vi "ADD Script-Completo.vi"(8 "error in (no error)":errorcluster, 9 "Datos a agregar":string, 11 "VISA resource name":refnum<visa-resource-name>) -> (0 "error out":errorcluster, 3 "VISA resource name out":refnum<visa-resource-name>)   [LabVIEW 2014, in "CAP-USB.lvlib"]
doc: "Genera el codigo para agregar una script\nal CAP-USB enviando todo el codigo por\nserie"
uses:
  CAP-USB.lvlib
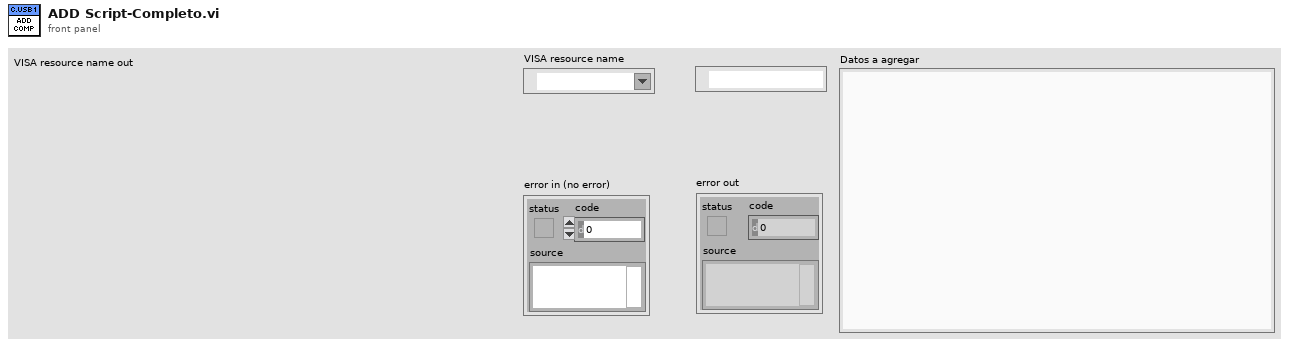
[diagram p1: front panel]
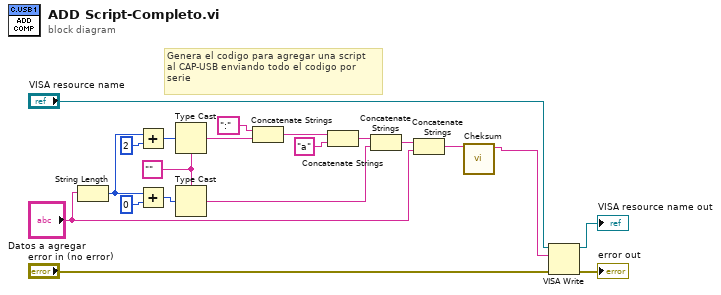
[diagram p0: block diagram]
diagram:
  w14 = "" ("COMANDO (a)")
  # "Genera el codigo para agregar una script\nal CAP-USB enviando todo el codigo por\nserie"
  n1 = String Length(string="Datos a agregar") -> (length=w8:i32)
  n2 = Add(x=w8, y=i8 2) -> (x+y=w15:i8)
  n3 = Add(x=w8, y=i8 0) -> (x+y=w6:i8)
  n4 = Type Cast(type=w14, x=w15) -> (*(type *) &x=w13:string)
  n5 = Type Cast(type=w14, x=w6) -> (*(type *) &x=w9:string)
  n6 = Concatenate Strings(":" ("COMANDO (a)"), w13) -> (w11:string)
  n7 = Concatenate Strings(w11, "a" ("COMANDO (a)")) -> (w18:string)
  n8 = Concatenate Strings(w18, w9) -> (w10:string)
  n9 = Concatenate Strings(w10, "Datos a agregar") -> (w2:string)
  n10 = call "Cheksum.vi"("Trama IN"=w2) -> ("Trama RTS"=w1:string)  [unwired: 9 in, 1 out]
  n11 = VISA Write(VISA resource name="VISA resource name", write buffer=w1, error in (no error)="error in (no error)") -> (VISA resource name out=→"VISA resource name out":refnum<visa-resource-name>, error out=→"error out":errorcluster)  [unwired: 1 out]
